vi "Write Prefix command.vi"(8 "error in (no error)":errorcluster, 10 "Prefix command":string, 11 "Keithley Meter in":refnum<class "Keithley Meter.lvclass">) -> (0 "error out":errorcluster, 3 "Keithley Meter out":refnum<class "Keithley Meter.lvclass">)   [LabVIEW 2015, in "Keithley Meter.lvclass"]
uses:
  Keithley Meter.lvclass
  Keithley Meter.lvclass/Keithley Meter.ctl
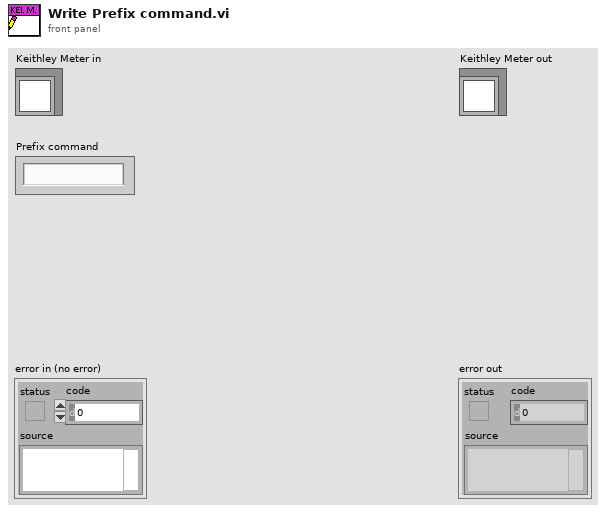
[diagram p1: front panel]
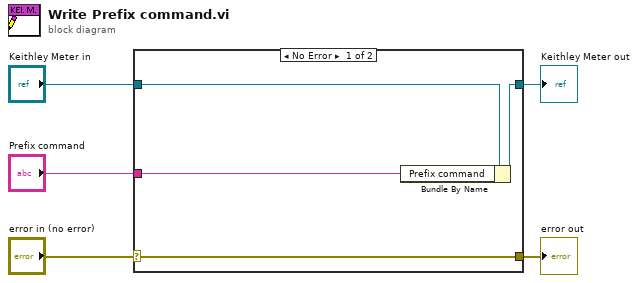
[diagram p0: block diagram]
diagram:
  n1 = case shown="No Error" "error in (no error)" {
    selector: "error in (no error)" -> [w9 w10]
    tunnel: [w9 w10] -> w4
    tunnel: [w7 w11] -> w2
    tunnel: "Keithley Meter in" -> [w8 w11]
    tunnel: "Prefix command" -> [w6 _]
    frame No Error {
      n2 = Bundle By Name(cluster=w8, "Prefix command"=w6) -> (w7:refnum<class "Keithley Meter.lvclass">)
    }
    frame Error {
    }
  }
  "error out" <- w4
  "Keithley Meter out" <- w2
